vi "Get Encoder State (uSMC).vi"(8 "error in (no error)":errorcluster, 10 "SMindex":i32, 11 "Visa array in":refnum<visa-resource-name>[](array[refnum])) -> (0 "error out":errorcluster, 1 "Encoder Current position":i32, 2 "Current Position in Encoder Units":i32, 3 "Visa array out":refnum<visa-resource-name>[](array[refnum]))   [LabVIEW 2010, in "SignalWriterMH110203USBStepperMotor.lvclass"]
uses:
  SignalWriterMH110203USBStepperMotor.lvclass
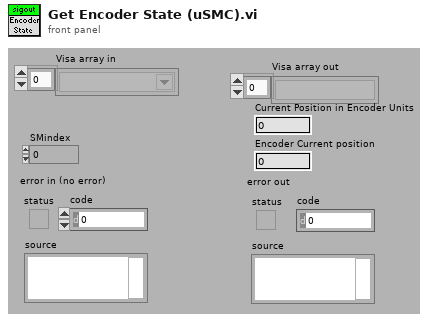
[diagram p1: front panel]
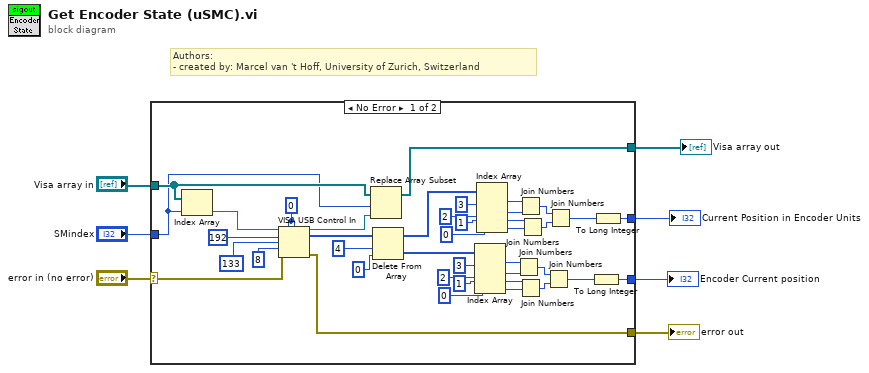
[diagram p0: block diagram]
diagram:
  # "Authors: \n- created by: Marcel van 't Hoff, University of Zurich, Switzerland"
  n1 = case shown="No Error" "error in (no error)" {
    selector: "error in (no error)" -> [w8 w49]
    tunnel: [w47 w49] -> w7
    tunnel: "Visa array in" -> [w40 w48]
    tunnel: "SMindex" -> [w38 _]
    tunnel: [w37 w48] -> w4
    tunnel: [w10 _] -> w3
    tunnel: [w9 _] -> w2
    frame No Error {
      w43 = u16 0 ("value (0)")
      n2 = Index Array(array=w40, index=w38) -> (element=w41:refnum<visa-resource-name>)
      n3 = VISA USB Control In(0:w41, 1:w43, 2:w43, 5:i16 192 ("request type"), 7:i16 133 ("request"), 9:u16 8 ("length (0)"), 11:w8) -> (4:w39:refnum<visa-resource-name>, 6:w42:u8[], 15:w47:errorcluster)
      n4 = Replace Array Subset(array=w40, new element=w39, index=w38) -> (w37:refnum<visa-resource-name>[])
      n5 = Delete From Array(array=w42, length=4, index=0) -> (deleted portion=w23:u8[], array with subset deleted=w11:u8[])
      n6 = Index Array(array=w23, index #1=3 ("index"), index #2=2 ("index"), index #3=1 ("index"), index #4=0 ("index")) -> (element #1=w29:u8, element #2=w30:u8, element #3=w28:u8, element #4=w27:u8)
      n7 = Index Array(array=w11, index #1=3 ("index"), index #2=2 ("index"), index #3=1 ("index"), index #4=0 ("index")) -> (element #1=w17:u8, element #2=w16:u8, element #3=w18:u8, element #4=w19:u8)
      n8 = Join Numbers(hi=w29, lo=w30) -> ((hi.lo)=w26:u16)
      n9 = Join Numbers(hi=w17, lo=w16) -> ((hi.lo)=w20:u16)
      n10 = Join Numbers(hi=w28, lo=w27) -> ((hi.lo)=w25:u16)
      n11 = Join Numbers(hi=w18, lo=w19) -> ((hi.lo)=w21:u16)
      n12 = Join Numbers(hi=w26, lo=w25) -> ((hi.lo)=w24:u32)
      n13 = Join Numbers(hi=w20, lo=w21) -> ((hi.lo)=w22:u32)
      n14 = To Long Integer(number=w24) -> (32bit integer=w9:i32)
      n15 = To Long Integer(number=w22) -> (32bit integer=w10:i32)
    }
    frame Error {
    }
  }
  "error out" <- w7
  "Visa array out" <- w4
  "Current Position in Encoder Units" <- w3
  "Encoder Current position" <- w2
